vi "带索引顺序排列-DBL.vi"(8 "排序模式":enum16{"从小到大", "从大到小"}(ring), 11 "数组":dbl[](array[numeric])) -> (0 "索引映射":i32[](array[numeric]), 3 "排序后":dbl[](array[numeric]))   [LabVIEW 2013]
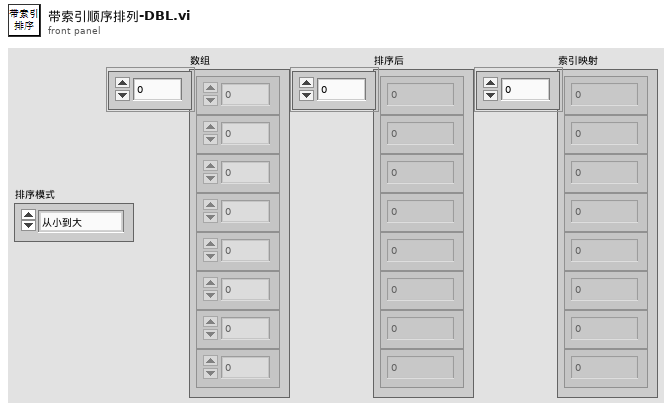
[diagram p1: front panel]
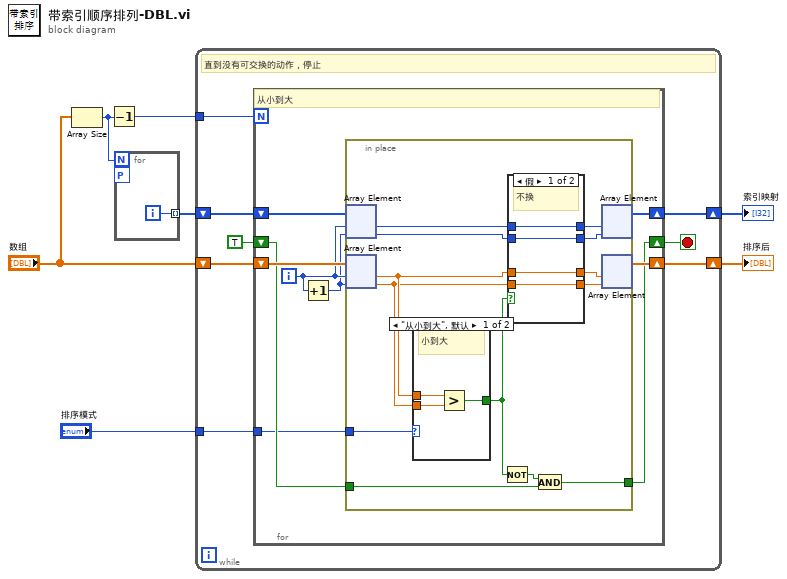
[diagram p0: block diagram]
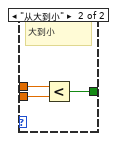
[diagram p2: hidden frame]
diagram:
  n1 = Array Size(array="数组") -> (size(s)=w5:i32)
  n2 = Decrement(x=w5) -> (x-1=w4:i32)
  n3 = for {
    N: w5 -> [_]
    workers-P: _ -> [_]
    tunnel: [w8] -> w7 mode=indexing
    i -> [w8]
  }
  n4 = while {
    tunnel: w4 -> [w14]
    shift-right: [w11] -> w1
    shift-left: "数组" -> [w16]
    shift-right: [w10] -> w2
    shift-left: w7 -> [w15]
    tunnel: "排序模式" -> [w9]
    stop <- w12 stop-if-true
    # "直到没有可交换的动作，停止"
    n5 = for {
      N: w14 -> [_]
      shift-right: [w24] -> w11
      shift-left: w16 -> [w25]
      shift-right: [w22] -> w10
      shift-left: w15 -> [w23]
      shift-right: [w21] -> w12
      shift-left: TRUE -> [w20]
      tunnel: w9 -> [w17]
      i -> [w19]
      # "从小到大"
      n6 = Increment(x=w19) -> (x+1=w18:i32)
      n7 = in-place {
        in-place-border: [w27] -> w21
        in-place-border: w20 -> [w28]
        in-place-border: w17 -> [w26]
        n8 = in-place-array #1(w23, w19, w18) -> (w33:i32, w31:i32)
        n9 = in-place-array #2(w25, w19, w18) -> (w37:dbl, w35:dbl)
        n10 = case shown="\"从小到大\", 默认" w26 {
          tunnel: w37 -> [w41 w44]
          tunnel: w35 -> [w40 w43]
          tunnel: [w39 w42] -> w30
          frame "从小到大", Default {
            # "小到大"
            n11 = Greater?(x=w41, y=w40) -> (0:w39:bool)
          }
          frame "从大到小" {
            # "大到小"
            n12 = Less?(x=w44, y=w43) -> (x < y?=w42:bool)
          }
        }
        n13 = Not(x=w30) -> (.not. x?=w29:bool)
        n14 = case shown="假" w30 {
          tunnel: [w48 w51] -> w38
          tunnel: w37 -> [w48 w52]
          tunnel: [w47 w52] -> w36
          tunnel: w35 -> [w47 w51]
          tunnel: [w45 w50] -> w34
          tunnel: w33 -> [w46 w50]
          tunnel: [w46 w49] -> w32
          tunnel: w31 -> [w45 w49]
          frame False {
            # "不换"
          }
          frame True {
            # "换"
          }
        }
        n15 = And(x=w29, y=w28) -> (x .and. y?=w27:bool)
        n16 = in-place-array #1(w32, w34) -> (w22:i32[])  [unwired: 2 out]
        n17 = in-place-array #2(w38, w36) -> (w24:dbl[])  [unwired: 2 out]
      }
    }
  }
  "排序后" <- w1
  "索引映射" <- w2
